vi "Receive Message.vi"(7 "Mediated Asynchronous Actor in":refnum<class "Mediated Asynchronous Actor.lvclass">, 8 "error in (no error)":errorcluster, 10 "Message in":refnum<class "Message Interface.lvclass">) -> (0 "error out":errorcluster, 3 "Stop?":bool, 5 "Mediated Asynchronous Actor out":refnum<class "Mediated Asynchronous Actor.lvclass">)   [LabVIEW 2016, in "Stream Mediator.lvlib" / "Mediated Asynchronous Actor.lvclass"]
doc: "--\nCopyright © 2017 Composed SystemsI All rights reserved.\n\nAuthor: Jon McBee <jon.mcbee@composed.io>\n\nThis library is provided \"AS IS\" ,WITHOUT WARRANTIES OR\nCONDITIONS OF ANY KIND, either express or implied.\n\nComposed Systems -- composed.io\n\nStream 0.0.1.1\nJon McBee - Composed Systems\nCopyright (c) 2017, Composed Systems"
uses:
  <userlib>/Composed Systems/Stream/Mediator/Classes/Mediated Asynchronous Actor/Mediated Asynchronous Actor.lvclass
  C:/Program Files (x86)/National Instruments/LabVIEW 2016/user.lib/Composed Systems/Stream/Actor/Actor Class/Ancestral Actor.lvclass
  <userlib>/Composed Systems/Stream/Mediator/Classes/Message Interface/Message Interface.lvclass
  <userlib>/Composed Systems/Stream/Mediator/Classes/Message Command Interface/Command Message Interface.lvclass
  <userlib>/Composed Systems/Stream/Log/Application Log/Log Level.ctl
  <userlib>/Composed Systems/Stream/Log/Global Application Log/Global Application Log.lvclass
  <userlib>/Composed Systems/Stream/Log/Application Log/Application Log.lvclass
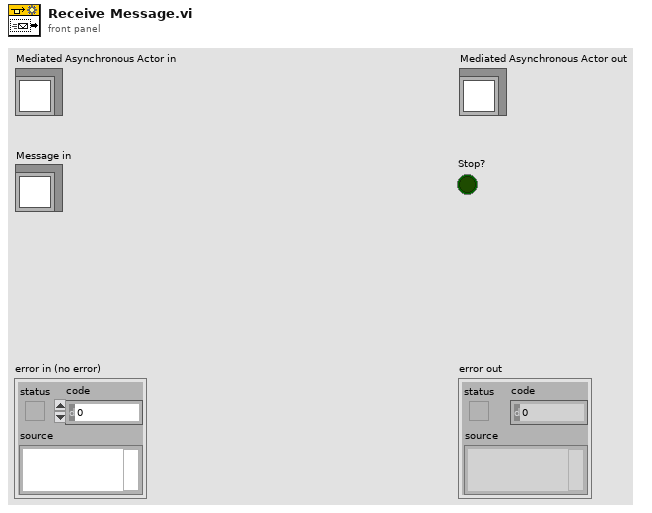
[diagram p1: front panel]
types:
  T1 = typedef "Stream Log.lvlib/Application Log.lvclass/Log Level.ctl" = enum16{"Imperative", "Major", "Minor", "Debug", "Off"}
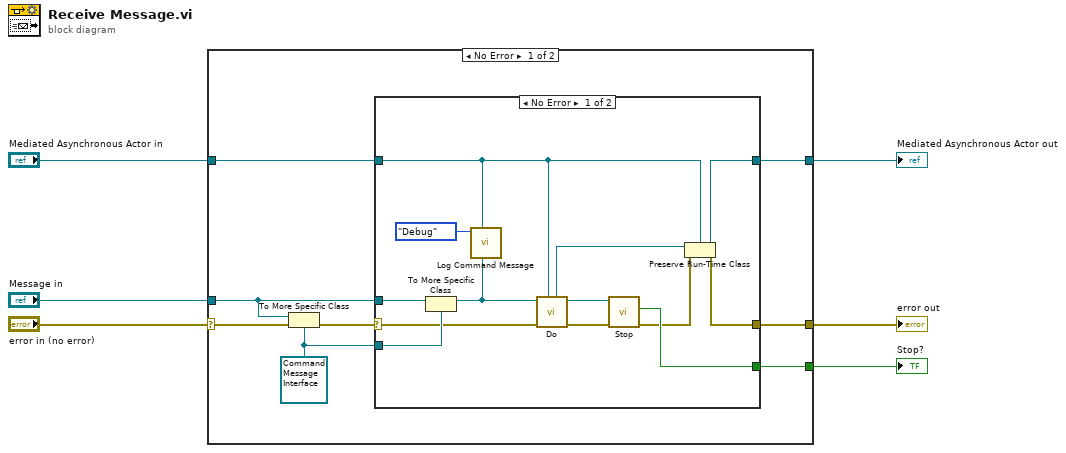
[diagram p0: block diagram]
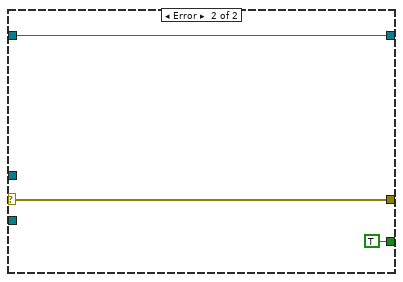
[diagram p2: hidden frame]
diagram:
  n1 = case shown="No Error" "error in (no error)" {
    selector: "error in (no error)" -> [w14 w32]
    tunnel: [w12 w32] -> w5
    tunnel: [w10 w31] -> w3
    tunnel: "Mediated Asynchronous Actor in" -> [w11 w31]
    tunnel: "Message in" -> [w7 _]
    tunnel: [w9 _] -> w1
    frame No Error {
      w8 = refnum<class "Command Message Interface.lvclass"> refnum ("Mediator Framework.lvlib:Command Message Interface.lvclass")
      n2 = To More Specific Class(target class=w8, reference=w7, error in=w14) -> (error out=w13:errorcluster)  [unwired: 1 out]
      n3 = case shown="No Error" w13 {
        selector: w13 -> [w23 w29]
        tunnel: [w18 w29] -> w12
        tunnel: [w15 w30] -> w10
        tunnel: w11 -> [w16 w30]
        tunnel: [w20 TRUE] -> w9
        tunnel: w8 -> [w26 _]
        tunnel: w7 -> [w27 _]
        frame No Error {
          n4 = To More Specific Class(target class=w26, reference=w27) -> (specific class reference=w22:refnum<class "Command Message Interface.lvclass">)  [unwired: 1 in, 1 out]
          n5 = call <userlib>:"Log Command Message.vi"("Command Message"=w22, "Actor"=w16, "Level"=Log_Level."Debug") -> ()  [unwired: 8 in, 1 out]
          n6 = call-dynamic "Do.vi"("Mediated Asynchronous Actor"=w16, "error in (no error)"=w23, "Command Message Interface in"=w22) -> ("error out"=w24:errorcluster, "Command Message Interface out"=w21:refnum<class "Command Message Interface.lvclass">, "Mediated Asynchronous Actor out"=w17:refnum<class "Mediated Asynchronous Actor.lvclass">)  [unwired: 6 in]
          n7 = call-dynamic "Stop.vi"("error in (no error)"=w24, "Command Message Interface in"=w21) -> ("error out"=w19:errorcluster, "Stop?"=w20:bool)  [unwired: 7 in, 1 out]
          n8 = Preserve Run-Time Class(object in=w17, error in=w19, 2:w16) -> (object out=w15:refnum<class "Mediated Asynchronous Actor.lvclass">, error out=w18:errorcluster)
        }
        frame Error {
        }
      }
    }
    frame Error {
    }
  }
  "error out" <- w5
  "Mediated Asynchronous Actor out" <- w3
  "Stop?" <- w1
